vi "InitDL.vi"(3 "Container State":T4 caption="État du conteneur", 4 "Previous State":variant caption="État précédent", 5 "Previous Version":T3 caption="Version précédente") -> (2 "Current State":T1={"Cells_VD2"=enum."5", "position"=0.0, "DS param"={"Domain name"="manip", "experiment"="VD2", "Device Server name"="DLs_VD2", "DL param"={"real pos"=-137.0, "max"=-30.0, "min"=120.0}, "preset pos"=[]}, "event"=refnum} caption="État actuel")   [LabVIEW 2020, in "OWIS_DLs_h.xctl"]
uses:
  OWIS_DLs_h.xctl
  stateDL.ctl
  controls/CellsSDI.ctl
  controls/CellBoolean.ctl
  <vilib>/_xctls/Container State.ctl
  <vilib>/_xctls/Version.ctl
  <vilib>/_xctls/XControlSupport.lvlib
panel:
  in  "Default Indicator State":T1={"Cells_VD2"=enum."5", "position"=0.0, "DS param"={"Domain name"="manip", "experiment"="VD2", "Device Server name"="DLs_VD2", "DL param"={"real pos"=-137.0, "max"=-30.0, "min"=120.0}, "preset pos"=[]}, "event"=refnum} caption="État de l'indicateur par défaut"
  in  "Default Control State":T1={"Cells_VD2"=enum."5", "position"=0.0, "DS param"={"Domain name"="manip", "experiment"="VD2", "Device Server name"="DLs_VD2", "DL param"={"real pos"=-137.0, "max"=-30.0, "min"=120.0}, "preset pos"=[]}, "event"=refnum} caption="État de la commande par défaut"
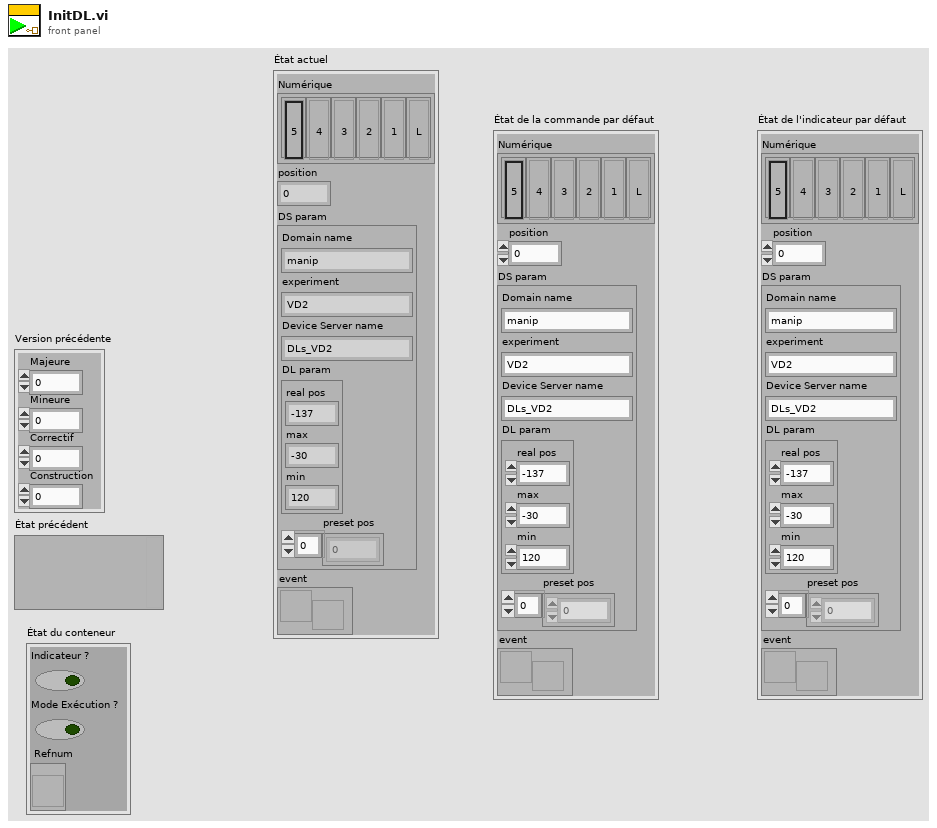
[diagram p1: front panel]
types:
  T1 = typedef "OWIS_DLs_h.xctl/stateDL.ctl" = cluster{"Cells_VD2":T2, "position":dbl, "DS param":cluster{"Domain name":string, "experiment":string, "Device Server name":string, "DL param":cluster{"real pos":dbl, "max":dbl, "min":dbl}, "preset pos":dbl[]}, "event":refnum<user-event>}
  T2 = typedef "CellsSDI.ctl" = enum32{"5", "4", "3", "2", "1", "L"}
  T3 = typedef "XControlSupport.lvlib/Version.ctl" = cluster{"Major":u16, "Minor":u16, "Fix":u16, "Build":u16}
  T4 = typedef "XControlSupport.lvlib/Container State.ctl" = cluster{"Indicator?":bool, "Run Mode?":bool, " Refnum":refnum<vi>}
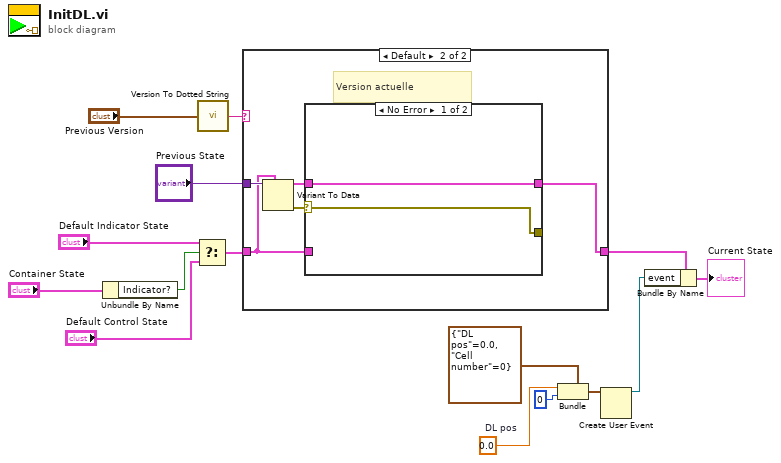
[diagram p0: block diagram]
diagram:
  w5 = 0.0  # DL pos
  n1 = Unbundle By Name("Container State") -> ("Indicator?"=w11:bool)
  n2 = Select(t="Default Indicator State", s=w11, f="Default Control State") -> (s? t:f=w10:T1)
  n3 = call <vilib>:"Version To Dotted String.vi"("Version"="Previous Version") -> ("String Version"=w8:string)
  n4 = case shown="Default" w8 {
    tunnel: "Previous State" -> [_ w21]
    tunnel: [w16 w17] -> w7
    tunnel: w10 -> [w16 w18]
    frame "0.0.0.0" {
      # "Nouvelle création ; utilisez l'état par défaut"
    }
    frame Default {
      # "Version actuelle"
      n5 = Variant To Data(type=w18, Variant=w21) -> (data=w19:T1, error out=w20:errorcluster)  [unwired: 1 in]
      n6 = case shown="No Error" w20 {
        selector: w20 -> [w23 w24]
        tunnel: w19 -> [w22 _]
        tunnel: [w22 w25] -> w17
        tunnel: w18 -> [_ w25]
        tunnel: [w23 w24] -> _
        frame No Error {
        }
        frame Error {
          # "Erreur de conversion de l'état\nenregistré précédent. Utilisez la valeur par défaut."
        }
      }
    }
  }
  n7 = Bundle(cluster=cluster{"DL pos":dbl, "Cell number":i32} {"DL pos"=0.0, "Cell number"=0} ("output cluster"), "DL pos"=w5, "Cell number"=0) -> (w4:cluster{"DL pos":dbl, "Cell number":i32})
  n8 = Create User Event(user event datatype=w4) -> (user event=w2:refnum<user-event>)  [unwired: 1 in, 1 out]
  n9 = Bundle By Name(cluster=w7, "event"=w2) -> (→"Current State":T1)
